vi "SW_Gen_Draw_numbers_and_highllights.vi"(5 "Regions to mark selected":u16[](array[numeric]), 6 "Colors cluster":T1, 7 "Regions to mark set":u16[](array[numeric]), 8 "Input cluster of parameters":T2={"Amount of border segments"=8, "Border segments starting angle"=0, "Amount of midfield segments"=4, "Midfield segments starting angle"=0, "Midfield segments outer radius, mm"=60, "Amount of central segments"=1, "Center segment outer radius, mm"=30, "Diameter of the cage, mm"=180, "R-gap between segments, mm"=10} {"Diameter of the cage, mm" scale=20.0..250.0}, 9 "Cluster of image geometrical and scaling parameters":T3, 10 "Bounding rectangles":T4, 11 "Zones layout input":picture) -> (2 "Array of the segment to color correspondences":u32[][](array[numeric]), 3 "Zones layout output":picture)   [LabVIEW 2016]
panel:
  in  "Bigger bubble radius":i32=15
  in  "Bubble radius":i16=11
  in  "Font size":i16=18
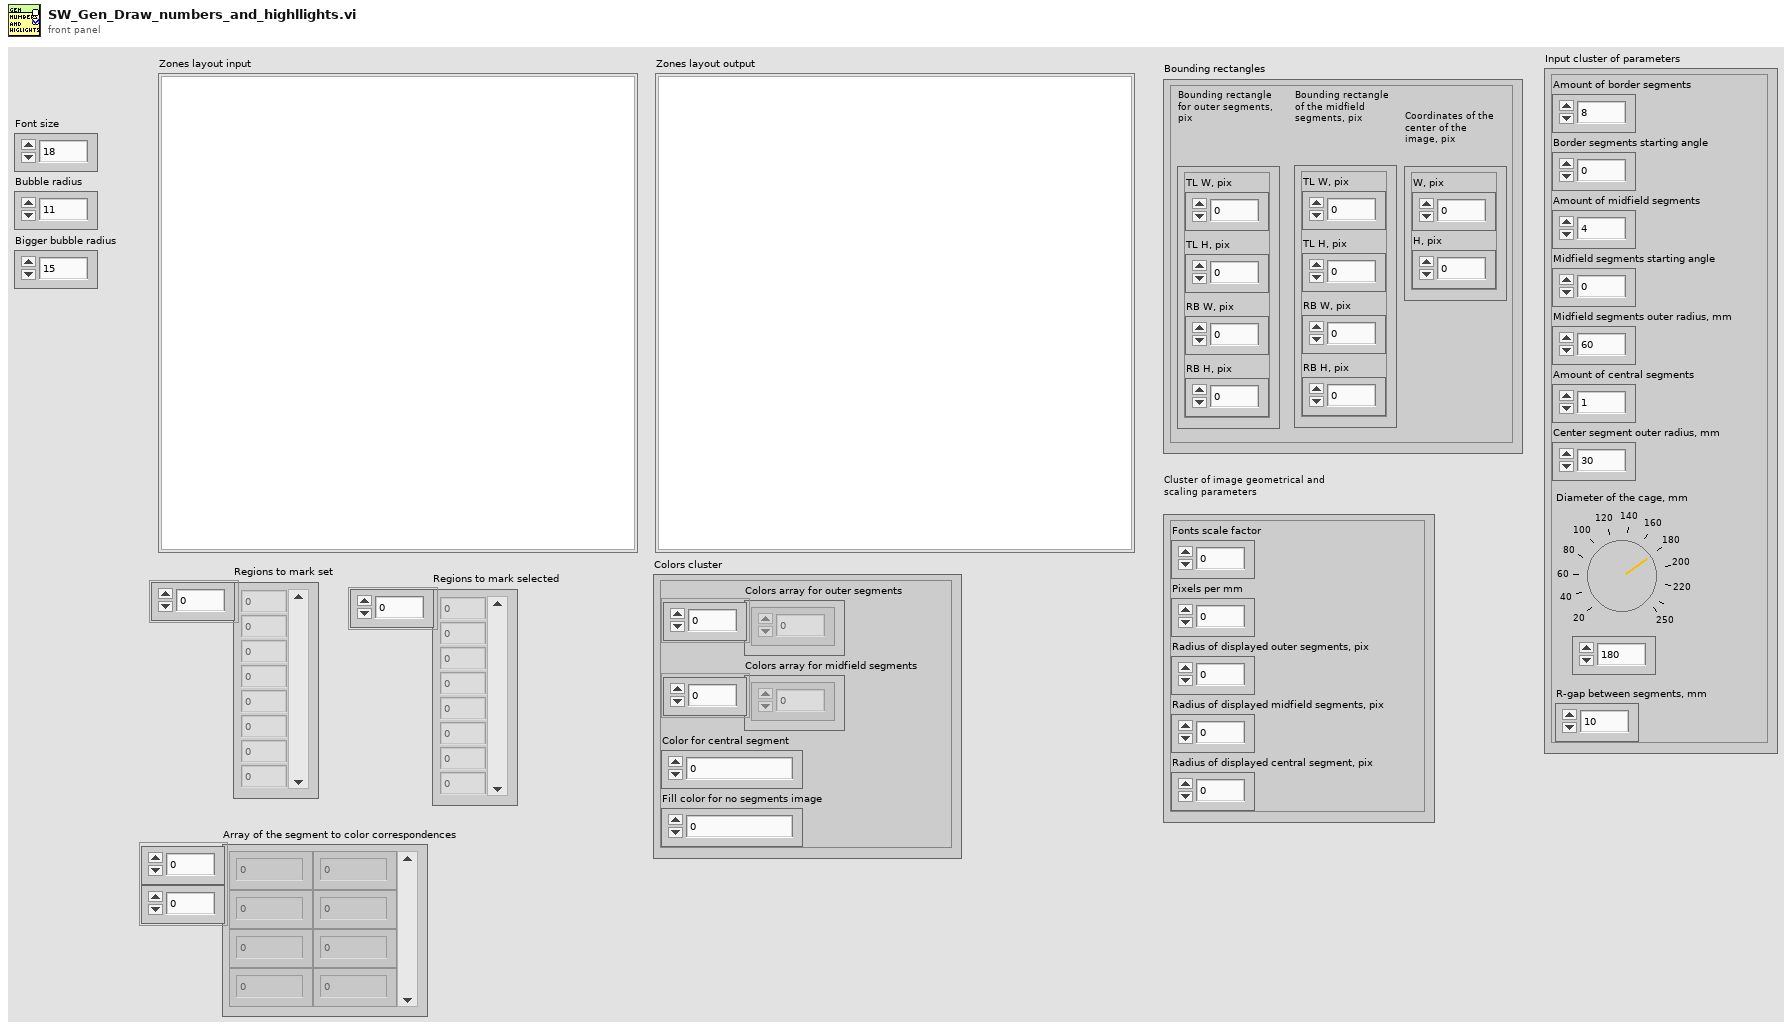
[diagram p1: front panel]
types:
  T1 = cluster{"Colors array for outer segments":u32[], "Colors array for midfield segments":u32[], "Color for central segment":u32, "Fill color for no segments image":u32}
  T2 = cluster{"Amount of border segments":u8, "Border segments starting angle":i16, "Amount of midfield segments":u8, "Midfield segments starting angle":i16, "Midfield segments outer radius, mm":u16, "Amount of central segments":u8, "Center segment outer radius, mm":u16, "Diameter of the cage, mm":u16, "R-gap between segments, mm":u8}
  T3 = cluster{"Fonts scale factor":dbl, "Pixels per mm":dbl, "Radius of displayed outer segments, pix":dbl, "Radius of displayed midfield segments, pix":dbl, "Radius of displayed central segment, pix":dbl}
  T4 = cluster{"Bounding rectangle for outer segments, pix":cluster{"TL W, pix":dbl, "TL H, pix":dbl, "RB W, pix":dbl, "RB H, pix":dbl}, "Bounding rectangle of the midfield segments, pix":cluster{"TL W, pix":dbl, "TL H, pix":dbl, "RB W, pix":dbl, "RB H, pix":dbl}, "Coordinates of the center of the image, pix":cluster{"W, pix":dbl, "H, pix":dbl}}
  T5 = enum16{"User-specified Font", "Application Font", "System Font", "Dialog Font"}
  T6 = cluster{"horizontal":enum16{"left", "center", "right"}, "vertical":enum16{"top", "center", "bottom"}}
  T7 = cluster{"TL W, pix":dbl, "TL H, pix":dbl, "RB W, pix":dbl, "RB H, pix":dbl}
  T8 = cluster{"Font Name:":string, "Size":i16, "Strikeout?":bool, "Italic?":bool, "Underline?":bool, "Outline?":bool, "Shadow?":bool, "Bold?":bool}
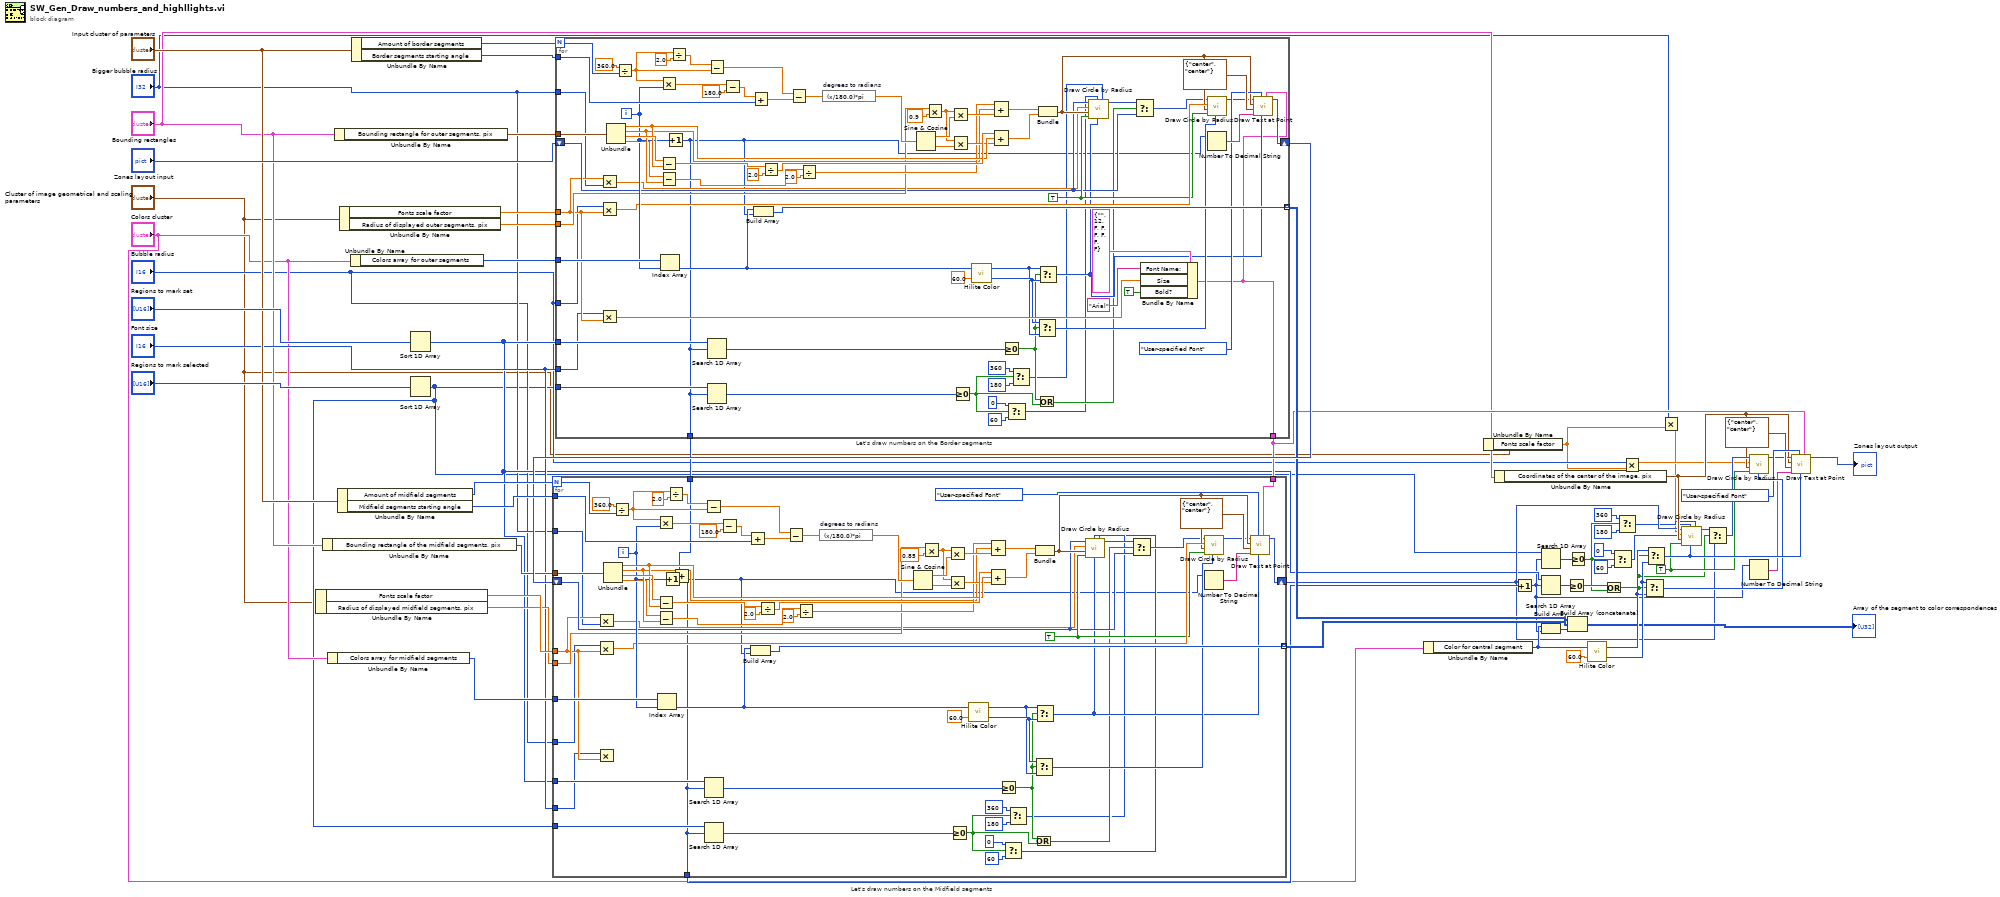
[diagram p0: block diagram]
diagram:
  w39 = TRUE ("fill?(F)")
  n1 = Unbundle By Name("Cluster of image geometrical and scaling parameters") -> ("Fonts scale factor"=w49:dbl, "Radius of displayed midfield segments, pix"=w48:dbl)
  n2 = Unbundle By Name("Bounding rectangles") -> ("Bounding rectangle of the midfield segments, pix"=w50:T7)
  n3 = Unbundle By Name("Colors cluster") -> ("Colors array for midfield segments"=w47:u32[])
  n4 = Unbundle By Name("Bounding rectangles") -> ("Bounding rectangle for outer segments, pix"=w60:T7)
  n5 = Unbundle By Name("Input cluster of parameters") -> ("Amount of midfield segments"=w53:u8, "Midfield segments starting angle"=w52:i16)
  n6 = Unbundle By Name("Cluster of image geometrical and scaling parameters") -> ("Fonts scale factor"=w58:dbl, "Radius of displayed outer segments, pix"=w59:dbl)
  n7 = Unbundle By Name("Colors cluster") -> ("Colors array for outer segments"=w55:u32[])
  n8 = Unbundle By Name("Input cluster of parameters") -> ("Amount of border segments"=w57:u8, "Border segments starting angle"=w56:i16)
  n9 = Sort 1D Array(array="Regions to mark set") -> (sorted array=w18:u16[])
  n10 = Sort 1D Array(array="Regions to mark selected") -> (sorted array=w14:u16[])
  n11 = for "Let's draw numbers on the Border segments" {
    N: w57 -> [w138]
    tunnel: w56 -> [w139]
    shift-right: [w118] -> w51
    shift-left: "Zones layout input" -> [w87]
    tunnel: w60 -> [w133]
    tunnel: w55 -> [w107]
    tunnel: w59 -> [w104]
    tunnel: [w101] -> w28 mode=indexing
    tunnel: w18 -> [w94]
    tunnel: w58 -> [w79]
    tunnel: w14 -> [w78]
    tunnel: "Font size" -> [w68]
    tunnel: "Bubble radius" -> [w67]
    tunnel: "Bigger bubble radius" -> [w66]
    tunnel: [w65] -> w45
    tunnel: [w64] -> w26
    i -> [w106]
    w90 = TRUE ("fill?(F)")
    n12 = Multiply(x=w79, y=w66) -> (x*y=w89:dbl)
    n13 = Multiply(x=w67, y=w79) -> (x*y=w95:dbl)
    n14 = Multiply(x=w68, y=w79) -> (x*y=w96:dbl)
    n15 = Unbundle(w133) -> ("TL W, pix"=w127:dbl, "TL H, pix"=w120:dbl, "RB W, pix"=w132:dbl, "RB H, pix"=w119:dbl)
    n16 = Divide(x=360.0, y=w138) -> (x/y=w108:dbl)
    n17 = Multiply(x=w108, y=w106) -> (x*y=w112:dbl)
    n18 = Subtract(x=w132, y=w127) -> (x-y=w130:dbl)
    n19 = Subtract(x=w119, y=w120) -> (x-y=w122:dbl)
    n20 = Index Array(array=w107, index=w106) -> (element=w84:u32)
    n21 = Increment(x=w106) -> (x+1=w65:i32)
    n22 = Divide(x=w108, y=2.0) -> (x/y=w110:dbl)
    n23 = Subtract(x=w110, y=w108) -> (x-y=w109:dbl)
    n24 = Search 1D Array(1D array=w94, element=w65) -> (index of element=w93:i32)  [unwired: 1 in]
    n25 = Search 1D Array(1D array=w78, element=w65) -> (index of element=w77:i32)  [unwired: 1 in]
    n26 = Subtract(x=w112, y=180.0) -> (x-y=w113:dbl)
    n27 = Add(x=w113, y=w139) -> (x+y=w136:dbl)
    n28 = Build Array(w84, w65) -> (w101:u32[])
    n29 = Divide(x=w130, y=2.0) -> (x/y=w128:dbl)
    n30 = Subtract(x=w109, y=w136) -> (x-y=w135:dbl)
    n31 = Divide(x=w122, y=2.0) -> (x/y=w124:dbl)
    n32 = expression code="(x/180.0)*pi" "degrees to radians"(w135) -> (w134:dbl)
    n33 = Sine & Cosine(0:w134) -> (1:w121:dbl, 2:w131:dbl)
    n34 = Multiply(x=w104, y=0.9) -> (x*y=w103:dbl)
    n35 = Multiply(x=w103, y=w121) -> (x*y=w125:dbl)
    n36 = Multiply(x=w103, y=w131) -> (x*y=w126:dbl)
    n37 = Greater Or Equal To 0?(x=w77) -> (x >= 0?=w70:bool)
    n38 = call <vilib>:"Hilite Color.vi"("Percentage(30)"=60.0, "Color In"=w84) -> ("Shadow"=w83:u32, "Hilite"=w82:u32)
    n39 = Compound Arithmetic op=ADD(w124, w120, w125) -> (w114:dbl)
    n40 = Compound Arithmetic op=ADD(w128, w127, w126) -> (w115:dbl)
    n41 = Greater Or Equal To 0?(x=w93) -> (x >= 0?=w81:bool)
    n42 = Select(t=i16 0 ("t 2"), s=w70, f=i16 60 ("start angle(0)")) -> (s? t:f=w71:i16)
    n43 = Select(t=i16 360, s=w70, f=i16 180 ("arc size(360)")) -> (s? t:f=w74:i16)
    n44 = Or(x=w81, y=w70) -> (x .or. y?=w75:bool)
    n45 = Select(t=w83, s=w81, f=w82) -> (s? t:f=w80:u32)
    n46 = Bundle(w114, w115) -> (w91:cluster{dbl, dbl})  [unwired: 1 in]
    n47 = Select(t=w82, s=w81, f=w83) -> (s? t:f=w76:u32)
    n48 = call <vilib>:"Draw Circle by Radius.vi"("arc size(360)"=w74, "color(black)"=w76, "start angle(0)"=w71, "fill?(F)"=w90, "pixel center"=w91, "radius"=w89, "picture"=w87) -> ("new picture"=w92:picture)  [unwired: 4 in]
    n49 = Select(t=w92, s=w75, f=w87) -> (s? t:f=w86:picture)
    n50 = Bundle By Name(cluster=T8 {"Font Name:"="", "Size"=12, "Strikeout?"=FALSE, "Italic?"=FALSE, "Underline?"=FALSE, "Outline?"=FALSE, "Shadow?"=FALSE, "Bold?"=FALSE} ("[user-specified font]"), "Font Name:"="Arial", "Size"=w96, "Bold?"=TRUE) -> (w64:T8)
    n51 = call <vilib>:"Draw Circle by Radius.vi"("color(black)"=w80, "fill?(F)"=w90, "pixel center"=w91, "radius"=w95, "picture"=w86) -> ("new picture"=w85:picture)  [unwired: 6 in]
    n52 = Number To Decimal String(number=w65) -> (decimal integer string=w116:string)  [unwired: 1 in]
    n53 = call <vilib>:"Draw Text at Point.vi"("[user-specified font]"=w64, "text color(black)"=w76, "desired font(Application)"=T5."User-specified Font", "text"=w116, "alignment(left, top)"=T6 {"horizontal"=enum."center", "vertical"=enum."center"}, "origin"=w91, "picture"=w85) -> ("new picture"=w118:picture)  [unwired: 3 in, 1 out]
  }
  n54 = for "Let's draw numbers on the Midfield segments" {
    N: w53 -> [w213]
    tunnel: w52 -> [w214]
    shift-right: [w193] -> w19
    shift-left: w51 -> [w166]
    tunnel: w50 -> [w208]
    tunnel: w47 -> [w182]
    tunnel: w48 -> [w179]
    tunnel: [w176] -> w27 mode=indexing
    tunnel: w18 -> [w173]
    tunnel: w49 -> [w158]
    tunnel: w14 -> [w156]
    tunnel: "Font size" -> [w146]
    tunnel: "Bubble radius" -> [w145]
    tunnel: "Bigger bubble radius" -> [w144]
    tunnel: w45 -> [w143]
    tunnel: w26 -> [w142]
    tunnel: [w141] -> w25
    i -> [w181]
    w169 = TRUE ("fill?(F)")
    n55 = Multiply(x=w158, y=w144) -> (x*y=w168:dbl)
    n56 = Multiply(x=w145, y=w158) -> (x*y=w174:dbl)
    n57 = Multiply(x=w146, y=w158) -> ()  [unwired: 1 out]
    n58 = Unbundle(w208) -> ("TL W, pix"=w202:dbl, "TL H, pix"=w195:dbl, "RB W, pix"=w207:dbl, "RB H, pix"=w194:dbl)
    n59 = Divide(x=360.0, y=w213) -> (x/y=w183:dbl)
    n60 = Multiply(x=w183, y=w181) -> (x*y=w187:dbl)
    n61 = Subtract(x=w207, y=w202) -> (x-y=w205:dbl)
    n62 = Subtract(x=w194, y=w195) -> (x-y=w197:dbl)
    n63 = Index Array(array=w182, index=w181) -> (element=w163:u32)
    n64 = Increment(x=w181) -> (x+1=w157:i32)
    n65 = Divide(x=w183, y=2.0) -> (x/y=w185:dbl)
    n66 = Add(x=w143, y=w157) -> (x+y=w141:i32)
    n67 = Subtract(x=w185, y=w183) -> (x-y=w184:dbl)
    n68 = Search 1D Array(1D array=w173, element=w141) -> (index of element=w172:i32)  [unwired: 1 in]
    n69 = Search 1D Array(1D array=w156, element=w141) -> (index of element=w155:i32)  [unwired: 1 in]
    n70 = Subtract(x=w187, y=180.0) -> (x-y=w188:dbl)
    n71 = Add(x=w188, y=w214) -> (x+y=w211:dbl)
    n72 = Build Array(w163, w141) -> (w176:u32[])
    n73 = Divide(x=w205, y=2.0) -> (x/y=w203:dbl)
    n74 = Subtract(x=w184, y=w211) -> (x-y=w210:dbl)
    n75 = Divide(x=w197, y=2.0) -> (x/y=w199:dbl)
    n76 = expression code="(x/180.0)*pi" "degrees to radians"(w210) -> (w209:dbl)
    n77 = Sine & Cosine(0:w209) -> (1:w196:dbl, 2:w206:dbl)
    n78 = Multiply(x=w179, y=0.85) -> (x*y=w178:dbl)
    n79 = Multiply(x=w178, y=w196) -> (x*y=w200:dbl)
    n80 = Multiply(x=w178, y=w206) -> (x*y=w201:dbl)
    n81 = Greater Or Equal To 0?(x=w155) -> (x >= 0?=w148:bool)
    n82 = call <vilib>:"Hilite Color.vi"("Percentage(30)"=60.0, "Color In"=w163) -> ("Shadow"=w162:u32, "Hilite"=w161:u32)
    n83 = Compound Arithmetic op=ADD(w199, w195, w200) -> (w189:dbl)
    n84 = Compound Arithmetic op=ADD(w203, w202, w201) -> (w190:dbl)
    n85 = Greater Or Equal To 0?(x=w172) -> (x >= 0?=w160:bool)
    n86 = Select(t=i16 0 ("t 2"), s=w148, f=i16 60 ("start angle(0)")) -> (s? t:f=w149:i16)
    n87 = Select(t=i16 360, s=w148, f=i16 180 ("arc size(360)")) -> (s? t:f=w152:i16)
    n88 = Or(x=w160, y=w148) -> (x .or. y?=w153:bool)
    n89 = Select(t=w162, s=w160, f=w161) -> (s? t:f=w159:u32)
    n90 = Bundle(w189, w190) -> (w170:cluster{dbl, dbl})  [unwired: 1 in]
    n91 = Select(t=w161, s=w160, f=w162) -> (s? t:f=w154:u32)
    n92 = call <vilib>:"Draw Circle by Radius.vi"("arc size(360)"=w152, "color(black)"=w154, "start angle(0)"=w149, "fill?(F)"=w169, "pixel center"=w170, "radius"=w168, "picture"=w166) -> ("new picture"=w171:picture)  [unwired: 4 in]
    n93 = Select(t=w171, s=w153, f=w166) -> (s? t:f=w165:picture)
    n94 = call <vilib>:"Draw Circle by Radius.vi"("color(black)"=w159, "fill?(F)"=w169, "pixel center"=w170, "radius"=w174, "picture"=w165) -> ("new picture"=w164:picture)  [unwired: 6 in]
    n95 = Number To Decimal String(number=w141) -> (decimal integer string=w191:string)  [unwired: 1 in]
    n96 = call <vilib>:"Draw Text at Point.vi"("[user-specified font]"=w142, "text color(black)"=w154, "desired font(Application)"=T5."User-specified Font", "text"=w191, "alignment(left, top)"=T6 {"horizontal"=enum."center", "vertical"=enum."center"}, "origin"=w170, "picture"=w164) -> ("new picture"=w193:picture)  [unwired: 3 in, 1 out]
  }
  n97 = Unbundle By Name("Colors cluster") -> ("Color for central segment"=w21:u32)
  n98 = Unbundle By Name("Cluster of image geometrical and scaling parameters") -> ("Fonts scale factor"=w1:dbl)
  n99 = Unbundle By Name("Bounding rectangles") -> ("Coordinates of the center of the image, pix"=w23:cluster{"W, pix":dbl, "H, pix":dbl})
  n100 = Increment(x=w25) -> (x+1=w13:i32)
  n101 = Search 1D Array(1D array=w14, element=w13) -> (index of element=w15:i32)  [unwired: 1 in]
  n102 = Search 1D Array(1D array=w18, element=w13) -> (index of element=w37:i32)  [unwired: 1 in]
  n103 = Build Array(w21, w13) -> (w33:u32[])
  n104 = Greater Or Equal To 0?(x=w37) -> (x >= 0?=w42:bool)
  n105 = Build Array (concatenate)(w28, w27, w33) -> (→"Array of the segment to color correspondences":u32[][])
  n106 = Greater Or Equal To 0?(x=w15) -> (x >= 0?=w7:bool)
  n107 = call <vilib>:"Hilite Color.vi"("Percentage(30)"=60.0, "Color In"=w21) -> ("Shadow"=w41:u32, "Hilite"=w40:u32)
  n108 = Or(x=w42, y=w7) -> (x .or. y?=w12:bool)
  n109 = Select(t=i16 0 ("t 2"), s=w7, f=i16 60 ("start angle(0)")) -> (s? t:f=w5:i16)
  n110 = Select(t=i16 360, s=w7, f=i16 180 ("arc size(360)")) -> (s? t:f=w6:i16)
  n111 = Multiply(x="Bubble radius", y=w1) -> (x*y=w4:dbl)
  n112 = Select(t=w41, s=w12, f=w40) -> (s? t:f=w43:u32)
  n113 = Select(t=w40, s=w12, f=w41) -> (s? t:f=w44:u32)
  n114 = Multiply(x="Bigger bubble radius", y=w1) -> (x*y=w2:dbl)
  n115 = call <vilib>:"Draw Circle by Radius.vi"("arc size(360)"=w6, "color(black)"=w44, "start angle(0)"=w5, "fill?(F)"=w39, "pixel center"=w23, "radius"=w2, "picture"=w19) -> ("new picture"=w38:picture)  [unwired: 4 in]
  n116 = Select(t=w38, s=w12, f=w19) -> (s? t:f=w36:picture)
  n117 = call <vilib>:"Draw Circle by Radius.vi"("color(black)"=w43, "fill?(F)"=w39, "pixel center"=w23, "radius"=w4, "picture"=w36) -> ("new picture"=w30:picture)  [unwired: 6 in]
  n118 = Number To Decimal String(number=w13) -> (decimal integer string=w32:string)  [unwired: 1 in]
  n119 = call <vilib>:"Draw Text at Point.vi"("[user-specified font]"=w26, "text color(black)"=w44, "desired font(Application)"=T5."User-specified Font", "text"=w32, "alignment(left, top)"=T6 {"horizontal"=enum."center", "vertical"=enum."center"}, "origin"=w23, "picture"=w30) -> ("new picture"=→"Zones layout output":picture)  [unwired: 3 in, 1 out]
